vi "Planta.vi"(0 "x_k-1":dbl, 1 "x_k-2":dbl, 2 "y_k-1":dbl, 3 "y_k-2":dbl) -> (7 "y_k":dbl)   [LabVIEW 2018]
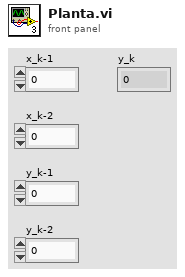
[diagram p1: front panel]
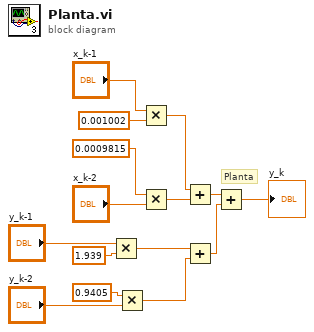
[diagram p0: block diagram]
diagram:
  # "Planta"
  n1 = Multiply(x="y_k-1", y=1.939) -> (x*y=w10:dbl)
  n2 = Multiply(x=0.9405, y="y_k-2") -> (x*y=w9:dbl)
  n3 = Multiply(x="x_k-1", y=0.001002) -> (x*y=w7:dbl)
  n4 = Multiply(x=0.0009815, y="x_k-2") -> (x*y=w8:dbl)
  n5 = Add(x=w7, y=w8) -> (x+y=w12:dbl)
  n6 = Add(x=w10, y=w9) -> (x+y=w11:dbl)
  n7 = Add(x=w12, y=w11) -> (x+y=→"y_k":dbl)
